vi "Config Data Registry.vi"(7 "function (get data)":T3=enum."get data" caption="Funktion (Daten lesen)", 8 "error in (no error)":errorcluster caption="Fehler (Eingang, kein Fehler)", 9 "section":string caption="Abschnitt", 10 "config data in":T4 caption="Konfigurationsdaten (Eingang)", 11 "config data":T2 caption="Konfigurationsdaten") -> (0 "error out":errorcluster caption="Fehler (Ausgang)", 1 "config data refnums":T2[](array[typedef]) caption="Konfigurationsdaten (RefNum)", 2 "config data out":T4 caption="Konfigurationsdaten (Ausgang)", 3 "config data out":T2 caption="Konfigurationsdaten (Ausgang)", 4 "valid index?":bool caption="Gültiger Index?", 5 "section":T1 caption="Abschnitt", 6 "valid section?":bool caption="Gültiger Abschnitt?")   [LabVIEW 2009]
doc: "Achtet auf die Daten die in Abhängigkeit mit dem Ojekt stehen. Die Funktionsparameter wird auf Objekte angewandt.\n\n* reset: Löscht und entfernt alle Objekte aus der Registry\n* Registrieren: Fügt ein Objekt zur Registry (Erzeugt einen Fehler wenn das Objekt schon vorhanden ist)\n* Hole Daten: Holt die Daten des Ojektes (Erzeugt einen Fehler wenn das Objekt nicht registriert ist)\n* Setze Daten: Setzt die Daten des Ojektes (Erzeugt einen Fehler wenn das Objekt nicht registriert ist)\n* Deregistrieren: Löscht und entfernt das Objekt aus der Registry (Erzeugt einen Fehler wenn das Objekt nicht registriert ist)\n* Hole Objekte: Gibt alle registrierten Objekte zurück"
uses:
  <vilib>/Utility/config.llb/Config Data RefNum.ctl
  Config Data.ctl
  Config Data Section.ctl
  Config Data Registry Functions.ctl
  <vilib>/Utility/config.llb/NI_LVConfig.lvlib
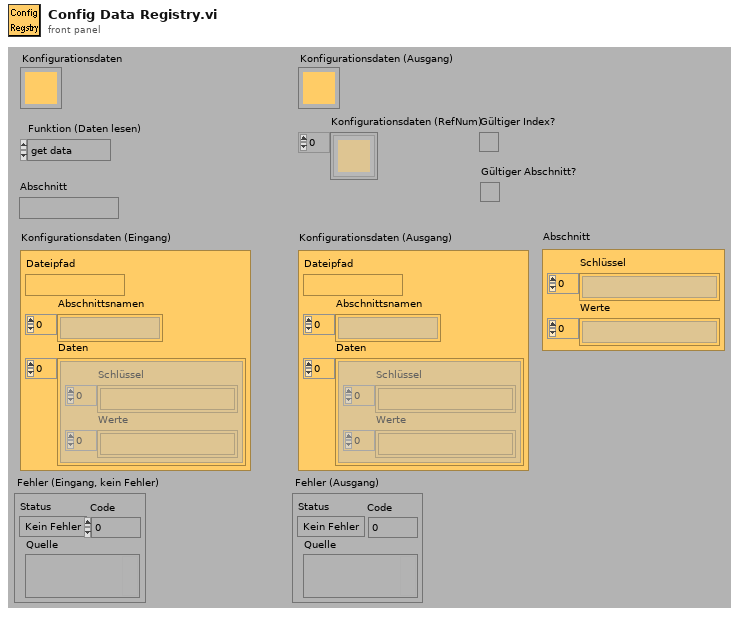
[diagram p1: front panel]
types:
  T1 = typedef "Config Data Section.ctl" = cluster{"keys":string[], "values":string[]}
  T2 = typedef "NI_LVConfig.lvlib/Config Data RefNum.ctl" = refnum<k1>
  T3 = typedef "Config Data Registry Functions.ctl" = enum16{"reset", "register", "get data", "get section", "set data", "unregister", "test", "get objects"}
  T4 = typedef "Config Data.ctl" = cluster{"file path":path, "data":T1[], "section names":string[]}
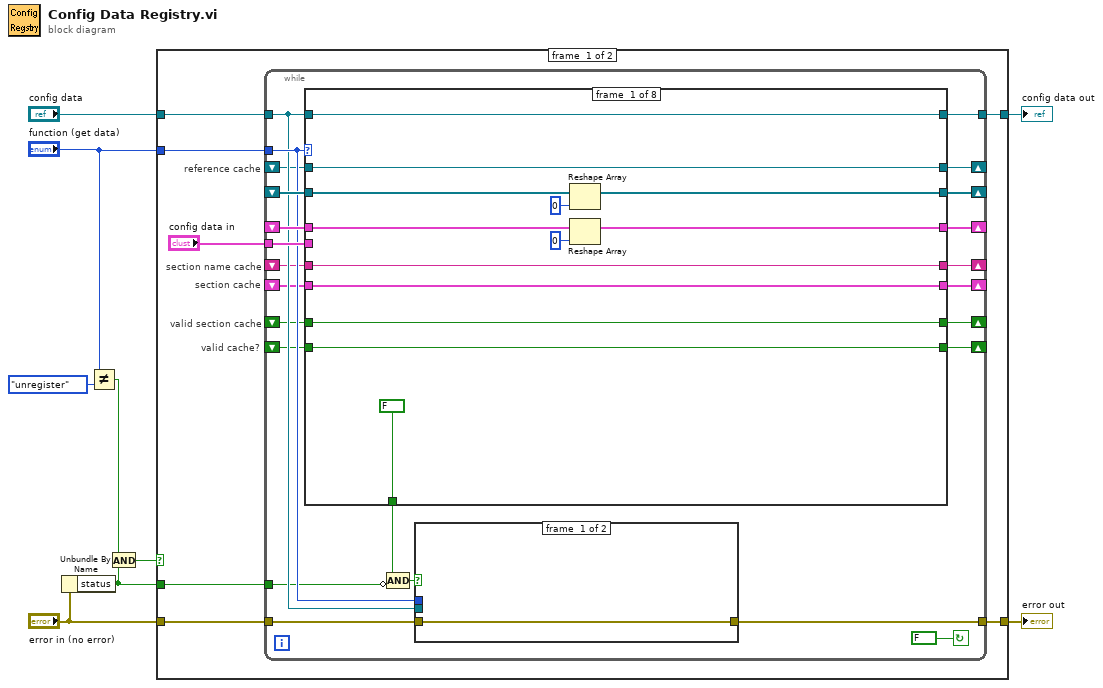
[diagram p0: block diagram]
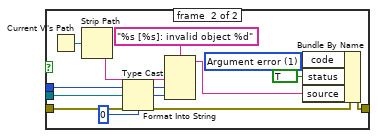
[diagram p2: hidden frame]
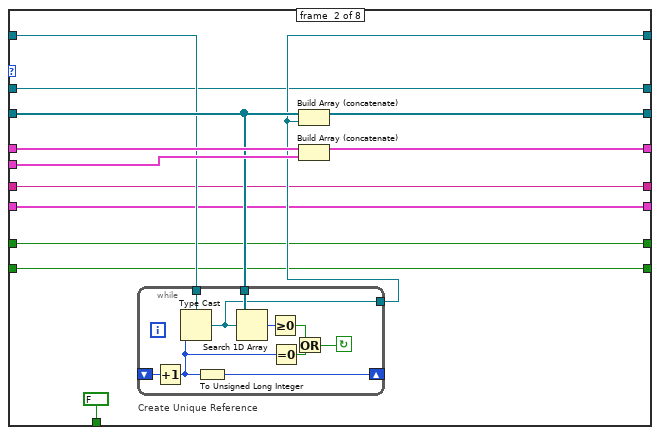
[diagram p3: hidden frame]
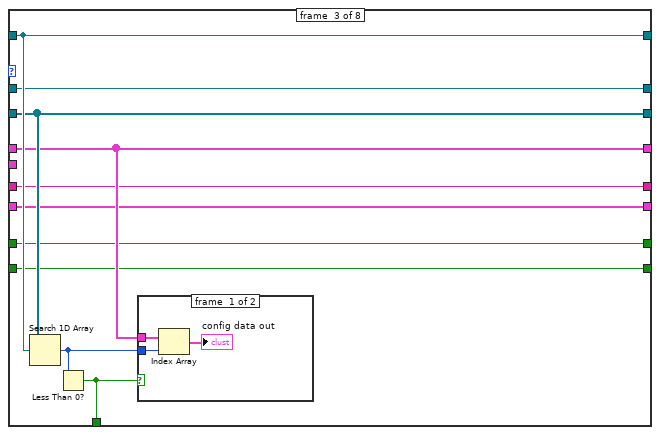
[diagram p4: hidden frame]
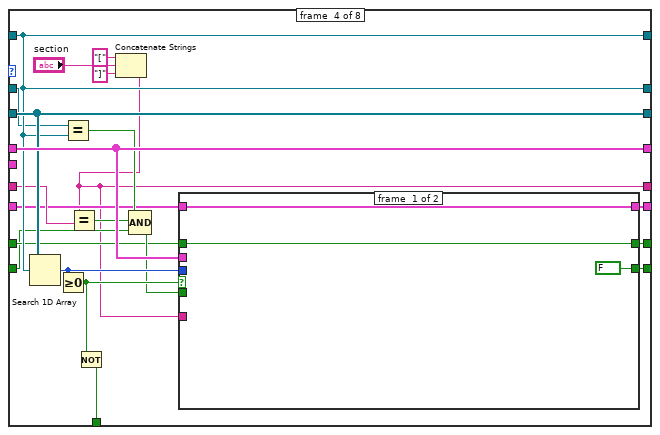
[diagram p6: hidden frame]
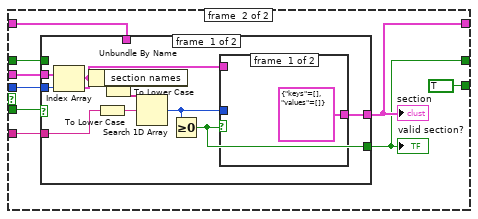
[diagram p7: hidden frame]
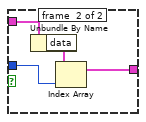
[diagram p8: hidden frame]
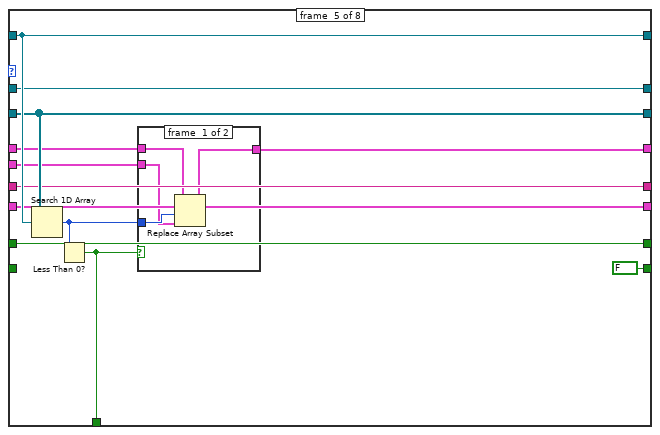
[diagram p10: hidden frame]
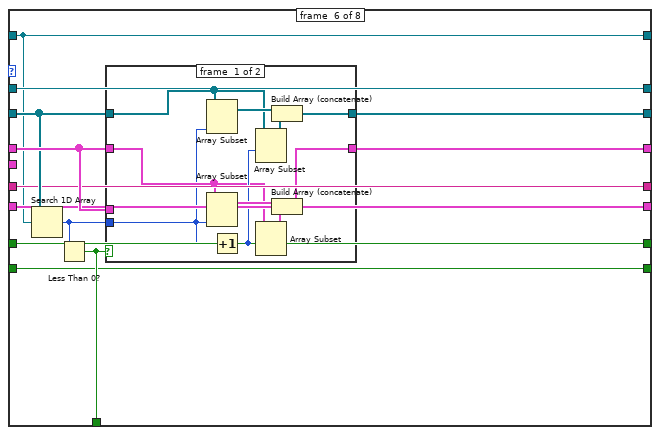
[diagram p12: hidden frame]
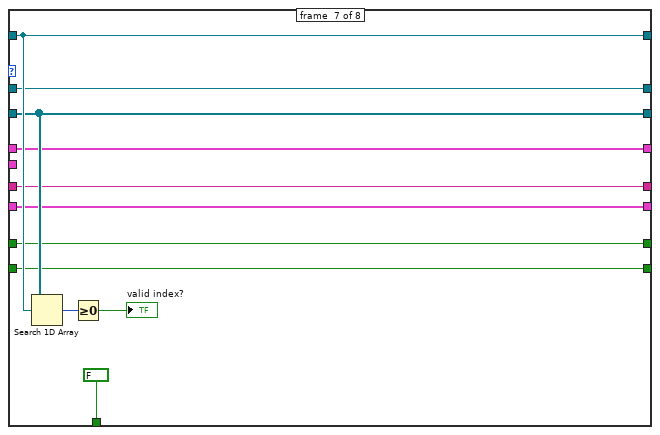
[diagram p14: hidden frame]
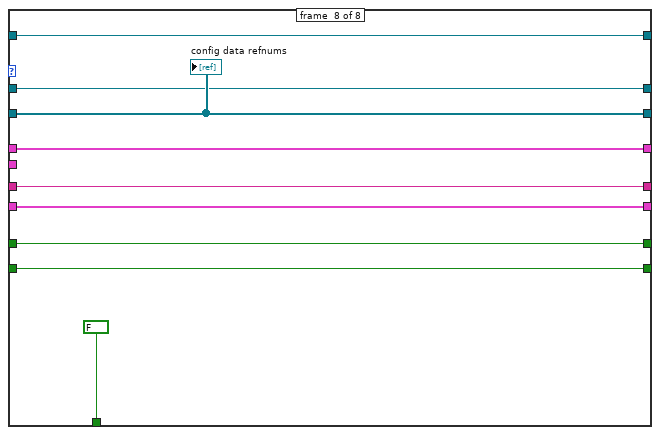
[diagram p15: hidden frame]
diagram:
  n1 = Unbundle By Name("error in (no error)") -> ("status"=w2:bool)
  n2 = Not Equal?(x="function (get data)", y=Config_Data_Registry_Functions."unregister" ("function (get data)")) -> (x != y?=w4:bool)
  n3 = And(x=w4, y=w2) -> (x .and. y?=w5:bool)
  n4 = case shown="False" w5 {
    tunnel: "error in (no error)" -> [w16 w215]
    tunnel: [w14 w214] -> w9
    tunnel: [w13 w215] -> w8
    tunnel: "config data" -> [w12 w214]
    tunnel: "function (get data)" -> [w11 _]
    tunnel: w2 -> [w10 _]
    frame #0 {
      # "valid cache?"
      # "valid section cache"
      # "section cache"
      # "section name cache"
      # "reference cache"
      n5 = while {
        shift-left: _ -> [w18]
        shift-right: [w19] -> _
        shift-left: _ -> [w21]
        shift-right: [w20] -> _
        shift-left: _ -> [w22]
        shift-right: [w23] -> _
        shift-left: _ -> [w24]
        shift-right: [w26] -> _
        shift-left: _ -> [w25]
        shift-right: [w27] -> _
        tunnel: w10 -> [w29]
        tunnel: [w31] -> w13
        tunnel: w16 -> [w32]
        tunnel: "config data in" -> [w35]
        tunnel: w11 -> [w34]
        tunnel: [w36] -> w14
        tunnel: w12 -> [w33]
        shift-left: _ -> [w38]
        shift-right: [w37] -> _
        shift-left: _ -> [w40]
        shift-right: [w39] -> _
        stop <- FALSE continue-if-true
        n6 = case shown="\"get section\"" w34 {
          tunnel: w40 -> [w59 w75 w98 w121 w163 w179 w202 w213]
          tunnel: w33 -> [w62 w73 w99 w119 w164 w171 w204 w211]
          tunnel: [w62 w72 w99 w119 w164 w171 w204 w211] -> w36
          tunnel: [w63 w79 w98 w121 w163 w178 w202 w213] -> w39
          tunnel: [w66 w77 w96 w122 w160 w177 w201 w212] -> w37
          tunnel: w38 -> [w60 w78 w96 w122 w161 w180 w201 w212]
          tunnel: w35 -> [_ w76 _ _ w159 _ _ _]
          tunnel: [FALSE FALSE w95 w111 w158 w176 FALSE FALSE] -> w30
          tunnel: [w58 w71 w94 w119 w157 w175 w198 w209] -> w27
          tunnel: [w57 w70 w93 w103 w156 w174 w197 w208] -> w26
          tunnel: w25 -> [w58 w71 w94 w118 w157 w175 w198 w209]
          tunnel: w24 -> [w57 w70 w93 w117 w156 w174 w197 w208]
          tunnel: [w56 w69 w92 w113 w155 w173 w196 w207] -> w23
          tunnel: w22 -> [w56 w69 w92 w112 w155 w173 w196 w207]
          tunnel: w21 -> [w55 w68 w91 w110 w154 w172 w195 w206]
          tunnel: [w55 w68 w91 w109 w154 w172 w195 w206] -> w20
          tunnel: [w54 w67 w90 w107 FALSE w170 w194 w205] -> w19
          tunnel: w18 -> [w54 w67 w90 w108 _ w170 w194 w205]
          frame #0 {
            n7 = Reshape Array(w59, 0) -> (w63:T2[])
            n8 = Reshape Array(w60, 0) -> (w66:T4[])
          }
          frame #1 {
            n9 = while "Create Unique Reference" {
              tunnel: [w80] -> w72
              tunnel: w75 -> [w84]
              tunnel: w73 -> [w85]
              shift-left: _ -> [w89]
              shift-right: [w88] -> _
              stop <- w81 continue-if-true
              n10 = Increment(x=w89) -> (x+1=w87:u32)
              n11 = Type Cast(type=w85, x=w87) -> (*(type *) &x=w80:T2)
              n12 = To Unsigned Long Integer(number=w87) -> (unsigned 32bit integer=w88:u32)
              n13 = Search 1D Array(1D array=w84, element=w80) -> (index of element=w86:i32)  [unwired: 1 in]
              n14 = Greater Or Equal To 0?(x=w86) -> (x >= 0?=w82:bool)
              n15 = Equal To 0?(x=w87) -> (x = 0?=w83:bool)
              n16 = Or(x=w82, y=w83) -> (x .or. y?=w81:bool)
            }
            n17 = Build Array (concatenate)(w75, w72) -> (w79:T2[])
            n18 = Build Array (concatenate)(w78, w76) -> (w77:T4[])
          }
          frame #2 {
            n19 = Search 1D Array(1D array=w98, element=w99) -> (index of element=w97:i32)  [unwired: 1 in]
            n20 = Less Than 0?(x=w97) -> (x < 0?=w95:bool)
            n21 = case shown="False" w95 {
              tunnel: w97 -> [w102 _]
              tunnel: w96 -> [w101 _]
              frame #0 {
                n22 = Index Array(array=w101, index=w102) -> (element=→"config data out":T4)
              }
              frame #1 {
              }
            }
          }
          frame #3 {
            n23 = Search 1D Array(1D array=w121, element=w119) -> (index of element=w123:i32)  [unwired: 1 in]
            n24 = Greater Or Equal To 0?(x=w123) -> (x >= 0?=w120:bool)
            n25 = Equal?(x=w118, y=w119) -> (x = y?=w116:bool)
            n26 = Not(x=w120) -> (.not. x?=w111:bool)
            n27 = Concatenate Strings("[", "section", "]") -> (w103:string)
            n28 = Equal?(x=w103, y=w117) -> (x = y?=w115:bool)
            n29 = Compound Arithmetic op=AND(w116, w115, w108) -> (w114:bool)
            n30 = case shown="True" w120 {
              tunnel: w123 -> [_ w135]
              tunnel: w122 -> [_ w134]
              tunnel: w103 -> [_ w133]
              tunnel: w114 -> [_ w132]
              tunnel: [w126 w131] -> w113
              tunnel: w112 -> [w126 w130]
              tunnel: w110 -> [w125 w128]
              tunnel: [w125 w129] -> w109
              tunnel: [FALSE TRUE] -> w107
              frame #0 {
              }
              frame #1 {
                n31 = case shown="False" w132 {
                  tunnel: w135 -> [w145 _]
                  tunnel: w134 -> [w144 _]
                  tunnel: w133 -> [w139 _]
                  tunnel: [w138 w152] -> w131
                  tunnel: w130 -> [_ w152]
                  tunnel: [w142 w151] -> w129
                  tunnel: w128 -> [_ w151]
                  frame #0 {
                    n32 = Index Array(array=w144, index=w145) -> (element=w141:T4)
                    n33 = Unbundle By Name(w141) -> ("section names"=w143:string[])
                    n34 = To Lower Case(string=w139) -> (all lower case string=w137:string)
                    n35 = To Lower Case(string=w143) -> (all lower case string=w136:string[])
                    n36 = Search 1D Array(1D array=w136, element=w137) -> (index of element=w140:i32)  [unwired: 1 in]
                    n37 = Greater Or Equal To 0?(x=w140) -> (x >= 0?=w142:bool)
                    n38 = case shown="True" w142 {
                      tunnel: w141 -> [_ w150]
                      tunnel: w140 -> [_ w148]
                      tunnel: [cluster{"keys":string[], "values":string[]} {"keys"=[], "values"=[]} ("section") w147] -> w138
                      frame #0 {
                      }
                      frame #1 {
                        n39 = Unbundle By Name(w150) -> ("data"=w149:T1[])
                        n40 = Index Array(array=w149, index=w148) -> (element=w147:T1)
                      }
                    }
                  }
                  frame #1 {
                  }
                }
                "section" <- w131
                "valid section?" <- w129
              }
            }
          }
          frame #4 {
            n41 = Search 1D Array(1D array=w163, element=w164) -> (index of element=w162:i32)  [unwired: 1 in]
            n42 = Less Than 0?(x=w162) -> (x < 0?=w158:bool)
            n43 = case shown="False" w158 {
              tunnel: w162 -> [w168 _]
              tunnel: w161 -> [w167 w169]
              tunnel: w159 -> [w166 _]
              tunnel: [w165 w169] -> w160
              frame #0 {
                n44 = Replace Array Subset(array=w167, new element=w166, index=w168) -> (w165:T4[])
              }
              frame #1 {
              }
            }
          }
          frame #5 {
            n45 = Search 1D Array(1D array=w179, element=w171) -> (index of element=w181:i32)  [unwired: 1 in]
            n46 = Less Than 0?(x=w181) -> (x < 0?=w176:bool)
            n47 = case shown="False" w176 {
              tunnel: w181 -> [w182 _]
              tunnel: w180 -> [_ _]
              tunnel: w180 -> [w183 w192]
              tunnel: w179 -> [w186 w193]
              tunnel: [w185 w193] -> w178
              tunnel: [w184 w192] -> w177
              frame #0 {
                n48 = Array Subset(array=w186, length=w182) -> (w188:T2[])  [unwired: 1 in]
                n49 = Array Subset(array=w183, length=w182) -> (w191:T4[])  [unwired: 1 in]
                n50 = Increment(x=w182) -> (x+1=w187:i32)
                n51 = Array Subset(array=w186, index=w187) -> (w189:T2[])  [unwired: 1 in]
                n52 = Array Subset(array=w183, index=w187) -> (w190:T4[])  [unwired: 1 in]
                n53 = Build Array (concatenate)(w188, w189) -> (w185:T2[])
                n54 = Build Array (concatenate)(w191, w190) -> (w184:T4[])
              }
              frame #1 {
              }
            }
          }
          frame #6 {
            n55 = Search 1D Array(1D array=w202, element=w204) -> (index of element=w203:i32)  [unwired: 1 in]
            n56 = Greater Or Equal To 0?(x=w203) -> (x >= 0?=→"valid index?":bool)
          }
          frame #7 {
            "config data refnums" <- w213
          }
        }
        n57 = Compound Arithmetic op=AND(w30, invert w29) -> (w28:bool)
        n58 = case shown="False" w28 {
          tunnel: w34 -> [_ w51]
          tunnel: w33 -> [_ w52]
          tunnel: w32 -> [w41 w46]
          tunnel: [w41 w45] -> w31
          frame #0 {
          }
          frame #1 {
            w42 = 1 items=["No error", "Argument error", "Memory is full", "Out of zone", "End of file", "File already open", "Generic file I/O error", "File not found", "File permission error", "Disk is full", "Duplicate path", "Too many files open", "System feature not enabled", "Resource file not found", "Cannot add resource", "Resource not found", "Image not found", "Image memory error", "Pen does not exist", "Config type invalid", "Config token not found", "Config parse error", "Config memory error", "Bad external code format", "Bad external code offset", "External code not present", "Null window", "Destroy window error", "Null menu", "Print aborted", "Bad print record", "Print driver error", "Windows error during printing", "Memory error during printing", "Print dialog error", "Generic print error", "Invalid device refnum", "Device not found", "Device parameter error", "Device unit error", "Cannot open device", "Device call aborted", "Generic error", "Cancelled by user", "Object ID too low", "Object ID too high", "Object not in heap", "Unknown heap", "Unknown object (invalid DefProc)", "Unknown object (DefProc not in table)", "Message out of range", "Invalid (null) method", "Unknown message", "Manager call not supported", "Bad address", "Network operation in progress", "Network operation timed out", "Connection is busy", "Network attribute not supported", "Network error", "Address in use", "System out of memory", "Connection aborted", "Connection refused", "Not connected", "Already connected", "Connection closed", "Initialization error (interapplication manager)", "Bad occurrence", "Wait on unbound occurrence handler", "Occurrence queue overflow", "Datalog type conflict", "Unused", "Unrecognized type (interapplication manager)", "Memory corrupt", "Failed to make temporary DLL", "Old CIN version", "Drag socket not found", "Failed to load drop-object", "Failed to register OLE object", "Failed to release OLE object", "Format specifier type mismatch", "Unknown format specifier", "Too few format specifiers", "Too many format specifiers", "Scan failed", "Newer CIN version", "Error converting to variant", "Runtime menu error", "Password tampered", "Variant attribute not found", "Incompatible variant data type", "Event data is not available", "Event Store is not present", "Occurrence is not found", "Event Queue is not created", "Event info is not available", "Refnum passed is NULL", "Error retrieving Class GUID", "Error retrieving CoClass GUID", "Error retrieving TypeLib GUID.", "Bad built application magic bytes.", "Specific driver is different from the specific driver associated with the Logical Name.", "There is no session opened to the class driver.", "Max Error", "MAX - Error with config objects", "MAX - Error loading configuration", "MAX - Group not supported"]
            n59 = Current VI's Path() -> (path=w50:path)
            n60 = Strip Path(path=w50) -> (name=w49:string)  [unwired: 1 out]
            n61 = Type Cast(type=u32 0 ("object"), x=w52) -> (*(type *) &x=w48:u32)
            n62 = Format Into String(format string="%s [%s]: invalid object %d", w49, w51, w48) -> (resulting string=w44:string)  [unwired: 2 in, 1 out]
            n63 = Bundle By Name(cluster=w46, "code"=w42, "status"=TRUE, "source"=w44) -> (w45:errorcluster)
          }
        }
      }
    }
    frame #1 {
    }
  }
  "config data out" <- w9
  "error out" <- w8
